vi "Curtin1_SelectCalib.vi"(9 "Save?":bool=TRUE, 11 "Settings in":T1={"Name of test"="", "Date"=timestamp(0 s since 1904-01-01), "Location"="", "Template"="", "Soundcard"="", "resolution"=32, "Sampling rate"=48000, "Ch1 Gain "=25.0, "Ch2 Gain"=10.0, "Sample time (s)"=0.3, "Pre-trigger (s)"=0.01, "Hammer Threshold"=10.0, "Positions"=12, "Taps/Position"=5, "Set Names"="", "Freq resolution"=10.0, "Hammer cutoff"=0.0, "Mic cutoff"=0.0, "Double bounce "=0.0, "Hammer Cal"=10.0, "dB Offset"=0.0, "Accel Cal"=10.0, "Vibrometer Cal"=0.0, "Mic Cal"=0.0, "Output"=2, "Voltage Cal"=0.01, "Vibrometer Port"="ASRL27::INSTR", "Range"=4, "High Pass"=2, "Bandwidth"=4, "X Range"=[], "Y Range"=[], "dB Spread"=0.0, "Trigger"=0, "Ch_1"=25, "Ch_2"=25, "flip?"=FALSE, "60Hz"=FALSE, "Time offset"=0.0, "Piezo Cal"=1.0, "Default Notes"=""} {"Ch_2" min=1 step=1; "Ch_1" min=1 max=100 step=1; "Trigger" items=["Hammer (force)", "Self-tap", "Spacebar"]; "Bandwidth" items=["1 kHz"=1, "5 kHz"=5, "10 kHz"=10, "25 kHz"=25, "50 kHz"=50, "100 kHz"=100]; "High Pass" items=["Off", "13 Hz", "104 Hz"]; "Range" items=["10 mm/s"=1, "20 mm/s"=2, "50 mm/s"=5, "100 mm/s"=10, "200 mm/s"=20, "500 mm/s"=50, "1 m/s"=100, "2 m/s"=200]; "Output" items=["Accelerometer", "Speed (from acceleration)", "Microphone", "Vibrometer", "Piezo"]; "Voltage Cal" format="%#_13g"; "Ch2 Gain" format="%#_13g"; "Ch1 Gain" format="%#_13g"; "Double bounce" min=0.0; "Mic cutoff" min=0.0 format="%#_4g"; "Hammer cutoff" min=0.0 format="%#_4g"; "Freq resolution" min=0.0; "Pre-trigger (s)" format="%#_13g"; "Date" format="%<%H:%M\n%d/%m/%y>T"; "resolution" items=["16 bit"=16, "24 bit"=24, "32 bit"=32]; "Sampling rate" items=["22050 samp/s"=22050, "44100 samp/s"=44100, "48000 samp/s"=48000]}) -> (3 "Settings out":T1={"Name of test"="", "Date"=timestamp(0 s since 1904-01-01), "Location"="", "Template"="", "Soundcard"="", "resolution"=32, "Sampling rate"=48000, "Ch1 Gain "=25.0, "Ch2 Gain"=10.0, "Sample time (s)"=0.3, "Pre-trigger (s)"=0.01, "Hammer Threshold"=10.0, "Positions"=12, "Taps/Position"=5, "Set Names"="", "Freq resolution"=10.0, "Hammer cutoff"=0.0, "Mic cutoff"=0.0, "Double bounce "=0.0, "Hammer Cal"=10.0, "dB Offset"=0.0, "Accel Cal"=10.0, "Vibrometer Cal"=0.0, "Mic Cal"=0.0, "Output"=2, "Voltage Cal"=0.01, "Vibrometer Port"="ASRL27::INSTR", "Range"=4, "High Pass"=2, "Bandwidth"=4, "X Range"=[], "Y Range"=[], "dB Spread"=0.0, "Trigger"=0, "Ch_1"=25, "Ch_2"=25, "flip?"=FALSE, "60Hz"=FALSE, "Time offset"=0.0, "Piezo Cal"=1.0, "Default Notes"=""} {"Ch_2" min=1 step=1; "Ch_1" min=1 max=100 step=1; "Trigger" items=["Hammer (force)", "Self-tap", "Spacebar"]; "Bandwidth" items=["1 kHz"=1, "5 kHz"=5, "10 kHz"=10, "25 kHz"=25, "50 kHz"=50, "100 kHz"=100]; "High Pass" items=["Off", "13 Hz", "104 Hz"]; "Range" items=["10 mm/s"=1, "20 mm/s"=2, "50 mm/s"=5, "100 mm/s"=10, "200 mm/s"=20, "500 mm/s"=50, "1 m/s"=100, "2 m/s"=200]; "Output" items=["Accelerometer", "Speed (from acceleration)", "Microphone", "Vibrometer", "Piezo"]; "Voltage Cal" format="%#_13g"; "Ch2 Gain" format="%#_13g"; "Ch1 Gain" format="%#_13g"; "Double bounce" min=0.0; "Mic cutoff" min=0.0 format="%#_4g"; "Hammer cutoff" min=0.0 format="%#_4g"; "Freq resolution" min=0.0; "Pre-trigger (s)" format="%#_13g"; "Date" format="%<%H:%M\n%d/%m/%y>T"; "resolution" items=["16 bit"=16, "24 bit"=24, "32 bit"=32]; "Sampling rate" items=["22050 samp/s"=22050, "44100 samp/s"=44100, "48000 samp/s"=48000]})   [LabVIEW 2022 SP3]
uses:
  PreferencesControl.ctl
panel:
  in  "Settings File":bool
  in  "delete":bool
  in  "Cancel Button":bool
  in  "OK Button":bool
  in  "Calib File":string(combo)
  # "Hz"
  # "dB"
  # "dB"
  # "sec"
  # "sec"
  # "mV/Pa"
  # "mV/m/s2"
  # "mV/mm/s"
  # "V/N"
  # "sec"
  # "sec"
  # "mV/N"
  # "a.u."
  # "a.u."
  # "sec"
  # "Hz"
  # "dB"
  # "dB"
  # "sec"
  # "sec"
  # "mV/Pa"
  # "mV/m/s2"
  # "mV/mm/s"
  # "V/N"
  # "sec"
  # "sec"
  # "mV/N"
  # "a.u."
  # "a.u."
  # "sec"
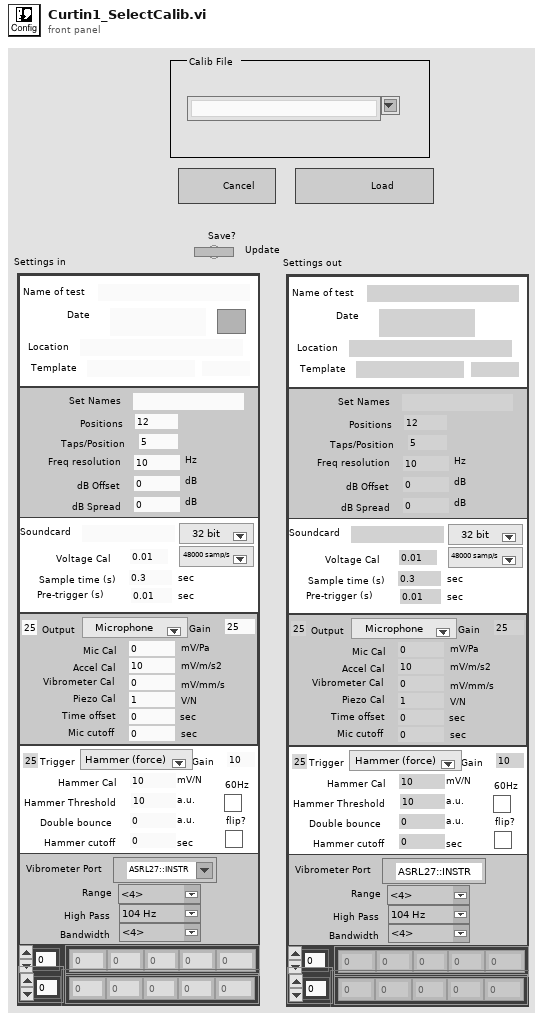
[diagram p1: front panel]
types:
  T1 = typedef "PreferencesControl.ctl" = cluster{"Name of test":string, "Date":timestamp, "Location":string, "Template":string, "Soundcard":string, "resolution":u16, "Sampling rate":u16, "Ch1 Gain ":dbl, "Ch2 Gain":dbl, "Sample time (s)":dbl, "Pre-trigger (s)":dbl, "Hammer Threshold":dbl, "Positions":i16, "Taps/Position":i16, "Set Names":string, "Freq resolution":dbl, "Hammer cutoff":dbl, "Mic cutoff":dbl, "Double bounce ":dbl, "Hammer Cal":dbl, "dB Offset":dbl, "Accel Cal":dbl, "Vibrometer Cal":dbl, "Mic Cal":dbl, "Output":u16, "Voltage Cal":dbl, "Vibrometer Port":refnum<visa-resource-name>, "Range":u16, "High Pass":u16, "Bandwidth":u16, "X Range":cluster{"Minimum":dbl, "Maximum":dbl, "Increment":dbl, "Minor Increment":dbl, "Start":dbl}[], "Y Range":cluster{"Minimum":dbl, "Maximum":dbl, "Increment":dbl, "Minor Increment":dbl, "Start":dbl}[], "dB Spread":dbl, "Trigger":u16, "Ch_1":u8, "Ch_2":u8, "flip?":bool, "60Hz":bool, "Time offset":dbl, "Piezo Cal":dbl, "Default Notes":string}
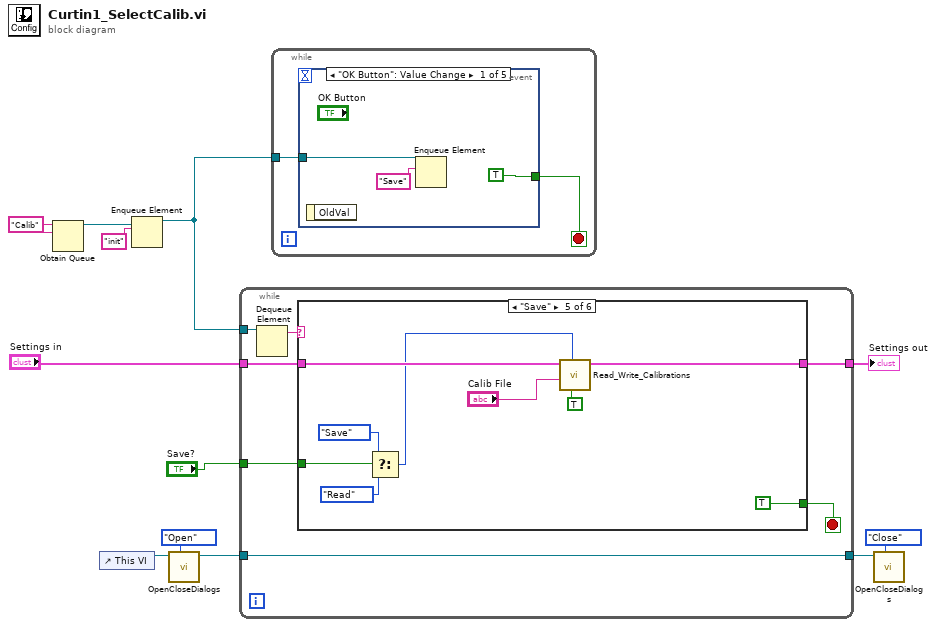
[diagram p0: block diagram]
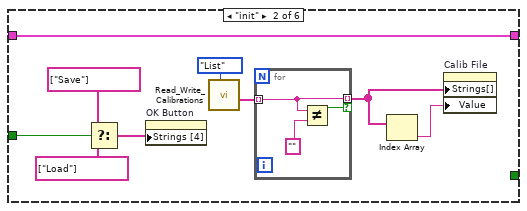
[diagram p3: hidden frame]
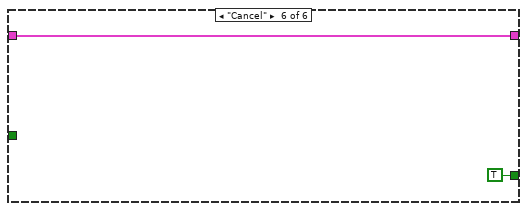
[diagram p6: hidden frame]
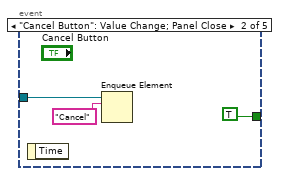
[diagram p7: hidden frame]
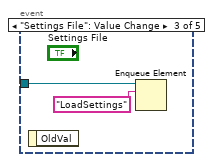
[diagram p8: hidden frame]
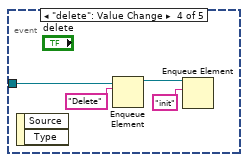
[diagram p9: hidden frame]
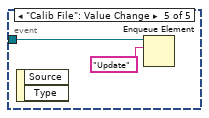
[diagram p10: hidden frame]
diagram:
  w12 = "Calib" ("name (unnamed)")
  n1 = Obtain Queue(name (unnamed)=w12, element data type=w12) -> (queue out=w11:refnum<queue>)  [unwired: 3 in, 2 out]
  n2 = control-ref of="This VI"() -> (w4:refnum<vi>)
  n3 = Enqueue Element(queue=w11, element="init") -> (queue out=w9:refnum<queue>)  [unwired: 2 in, 2 out]
  n4 = call "OpenCloseDialogs.vi"("Task"=enum16{"Open", "Close"}."Open", "VI in"=w4) -> ("VI out"=w2:refnum<vi>)  [unwired: 8 in, 1 out]
  n5 = while {
    tunnel: w9 -> [w18]
    tunnel: "Settings in" -> [w16]
    tunnel: [w15] -> w7
    tunnel: "Save?" -> [w14]
    tunnel: w2 -> [w13]
    tunnel: [w13] -> w1
    stop <- w17 stop-if-true
    n6 = Dequeue Element(queue=w18) -> (element=w19:string)  [unwired: 2 in, 3 out]
    n7 = case shown="\"Save\"" w19 {
      tunnel: [_ _ _ _ TRUE TRUE] -> w17
      tunnel: w16 -> [w20 w28 w33 w34 w42 w44]
      tunnel: [w20 w28 w33 w34 w40 w44] -> w15
      tunnel: w14 -> [_ w21 _ _ w39 _]
      frame Default {
      }
      frame "init" {
        n8 = Select(t=string[] ["Save"] ("Strings [4]"), s=w21, f=string[] ["Load"] ("Strings [4]")) -> (s? t:f=w23:string[])
        n9 = property on="OK Button" class="Bool"("Strings [4]"=w23) -> ()  [unwired: 2 in, 2 out]
        n10 = call "Read_Write_Calibrations.vi"("Task"=enum16{"Save", "Read", "List"}."List") -> ("Cal files"=w26:string[])  [unwired: 8 in, 2 out]
        n11 = for {
          tunnel: w26 -> [w30] mode=indexing
          tunnel: [w30] -> w29 mode=indexing if=w32
          n12 = Not Equal?(x=w30, y="") -> (x != y?=w32:bool)
        }
        n13 = Index Array(array=w29) -> (element=w25:string)  [unwired: 1 in]
        n14 = property on="Calib File" class="CmbBox"("Strings[]"=w29, "Value"=w25) -> ()  [unwired: 2 in, 2 out]
      }
      frame "Delete" {
      }
      frame "Update" {
      }
      frame "Save" {
        n15 = Select(t=enum16{"Save", "Read", "List"}."Save" ("Task"), s=w39, f=enum16{"Save", "Read", "List"}."Read" ("Task")) -> (s? t:f=w36:enum16{"Save", "Read", "List"})
        n16 = call "Read_Write_Calibrations.vi"("Silent?"=TRUE, "Task"=w36, "Calibration name"="Calib File", "Settings in"=w42) -> ("Settings out"=w40:T1)  [unwired: 5 in, 2 out]
      }
      frame "Cancel" {
      }
    }
  }
  "Settings out" <- w7
  n17 = while {
    tunnel: w9 -> [w46]
    stop <- w47 stop-if-true
    n18 = event shown="[0] \"OK Button\": Value Change" {
      selector: _ -> [_ _ _ _ _]
      dyn-events: _ -> [_ _ _ _ _]
      timeout: _ -> [_ _ _ _ _]
      tunnel: [TRUE ("OK Button") TRUE ("OK Button") _ _ _] -> w47
      tunnel: w46 -> [w48 w51 w54 w58 w60]
      event "OK Button": Value Change {
        n19 = event-data() -> ()  [unwired: 1 in, 1 out]
        n20 = Enqueue Element(queue=w48, element="Save") -> ()  [unwired: 2 in, 3 out]
      }
      event "Cancel Button": Value Change; Panel Close {
        n21 = event-data() -> ()  [unwired: 1 in, 1 out]
        n22 = Enqueue Element(queue=w51, element="Cancel") -> ()  [unwired: 2 in, 3 out]
      }
      event "Settings File": Value Change {
        n23 = event-data() -> ()  [unwired: 1 in, 1 out]
        n24 = Enqueue Element(queue=w54, element="LoadSettings") -> ()  [unwired: 2 in, 3 out]
      }
      event "delete": Value Change {
        n25 = event-data() -> ()  [unwired: 1 in, 2 out]
        n26 = Enqueue Element(queue=w58, element="Delete") -> (queue out=w56:refnum<queue>)  [unwired: 2 in, 2 out]
        n27 = Enqueue Element(queue=w56, element="init") -> ()  [unwired: 2 in, 3 out]
      }
      event "Calib File": Value Change {
        n28 = event-data() -> ()  [unwired: 1 in, 2 out]
        n29 = Enqueue Element(queue=w60, element="Update") -> ()  [unwired: 2 in, 3 out]
      }
    }
  }
  n30 = call "OpenCloseDialogs.vi"("Task"=enum16{"Open", "Close"}."Close", "VI in"=w1) -> ()  [unwired: 8 in, 2 out]
